vi "Dig PWM Meas Check for Multiple Global Channels.vi"(0 "Global Channel In":refnum<k21>, 11 "error in (no error)":errorcluster) -> (4 "Global Channel Out":refnum<k21>, 15 "error out":errorcluster)   [LabVIEW 2021, in "DAQ_Digital PWM Measurement.lvlib"]
doc: "Checks for the presence of multiple global channels and throws the error if identified"
uses:
  DAQ_Digital PWM Measurement.lvlib
  <vilib>/Utility/error.llb/Error Cluster From Error Code.vi
  <vilib>/ErrorRing/Error Ring.xnode
  <resource>/objmgr/daqmx.rc
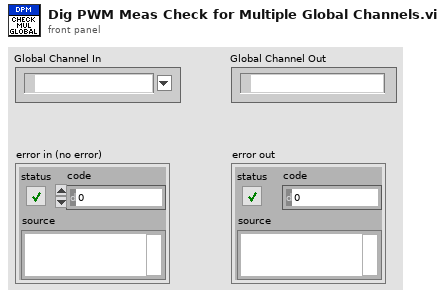
[diagram p1: front panel]
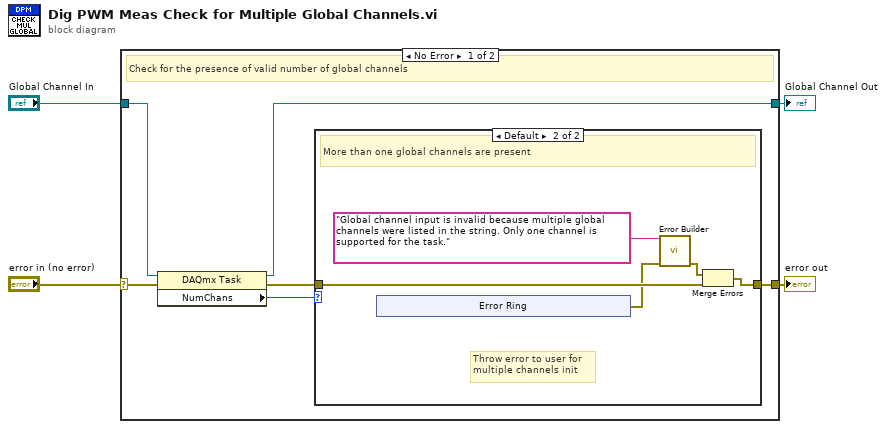
[diagram p0: block diagram]
diagram:
  n1 = case shown="No Error" "error in (no error)" {
    selector: "error in (no error)" -> [w8 w21]
    tunnel: "Global Channel In" -> [w7 w22]
    tunnel: [w6 w22] -> w2
    tunnel: [w5 w21] -> w1
    frame No Error {
      # "Check for the presence of valid number of global channels"
      n2 = property class="DAQmx Task"(reference=w7, error in=w8) -> (reference out=w6:refnum<k21>, error out=w10:errorcluster, "NumChans"=w9:u32)
      n3 = case shown="Default" w9 {
        tunnel: w10 -> [w11 w15]
        tunnel: [w11 w16] -> w5
        frame 1 {
          # "Only 1 channel is present (valid scenario)"
        }
        frame Default {
          # "Throw error to user for \nmultiple channels init"
          # "More than one global channels are present"
          n4 = xnode "Error Ring"() -> ("error out"=w14:errorcluster)
          n5 = call "Error Builder.vi"("Error String"="Global channel input is invalid because multiple global channels were listed in the string. Only one channel is supported for the task." ("error message (\"\")"), "Error In"=w14) -> ("Error Out"=w12:errorcluster)  [unwired: 13 in]
          n6 = Merge Errors(w12, w15) -> (w16:errorcluster)
        }
      }
    }
    frame Error {
      # "Error scenario - Do nothing"
    }
  }
  "error out" <- w1
  "Global Channel Out" <- w2
